vi "Add Protection.vi"(8 "error in (no error)":errorcluster, 9 "Pad":bool, 10 "String in":string, 11 "SMC Protection in":refnum<class "SMC Protection.lvclass">) -> (0 "error out":errorcluster, 2 "String out":string, 3 "SMC Protection out":refnum<class "SMC Protection.lvclass">)   [LabVIEW 2021, in "Protections.lvlib" / "SMC Protection.lvclass"]
uses:
  SMC Protection.lvclass
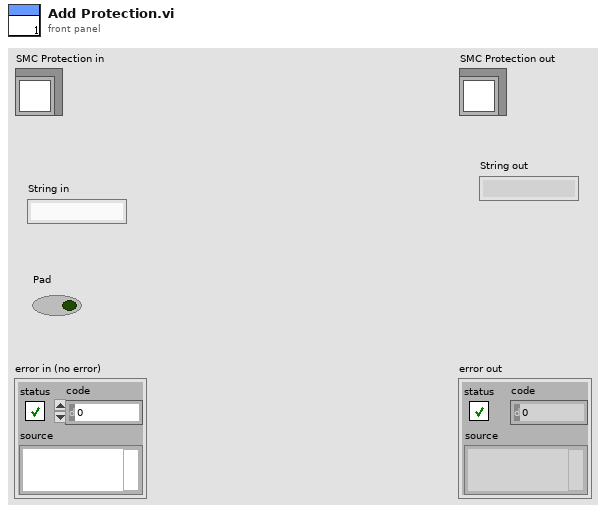
[diagram p1: front panel]
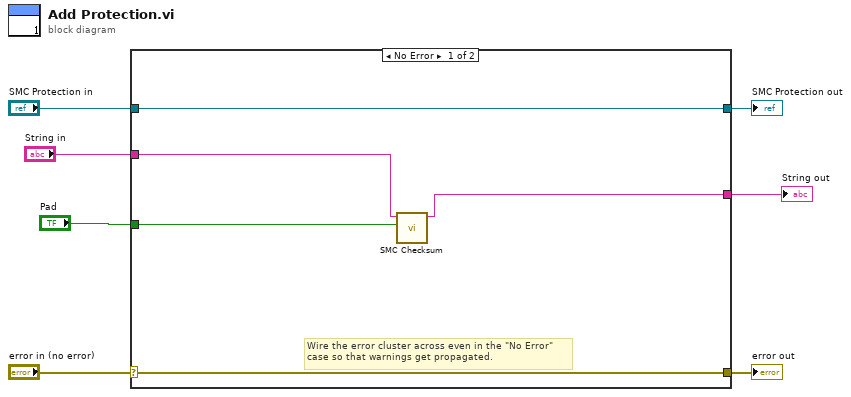
[diagram p0: block diagram]
diagram:
  n1 = case shown="No Error" "error in (no error)" {
    selector: "error in (no error)" -> [w11 w15]
    tunnel: [w11 w15] -> w6
    tunnel: [w12 w14] -> w4
    tunnel: "SMC Protection in" -> [w12 w14]
    tunnel: "Pad" -> [w10 _]
    tunnel: [w9 w13] -> w2
    tunnel: "String in" -> [w8 w13]
    frame No Error {
      # "Wire the error cluster across even in the \"No Error\"\ncase so that warnings get propagated."
      n2 = call "SMC Checksum.vi"("Pad"=w10, "String in"=w8) -> ("result string"=w9:string)  [unwired: 8 in, 1 out]
    }
    frame Error {
    }
  }
  "error out" <- w6
  "SMC Protection out" <- w4
  "String out" <- w2
